vi "ziSaveSettings.vi"(3 "Error In":errorcluster, 4 "Path (\"\")":string, 5 "file path (dialog if empty)":path, 6 "Handle In":T1 {"Handle" format="0x%08x"; "Conn" format="0x%08x"}) -> (0 "Error Out":errorcluster, 1 "Saved Array":string[][](array[string]), 2 "Handle Out":T1 {"Handle" format="0x%08x"; "Conn" format="0x%08x"})   [LabVIEW 2009, in "Zurich Instruments LabOne.lvlib"]
uses:
  <instrlib>/Zurich Instruments LabOne/Zurich Instruments LabOne.lvlib
  <instrlib>/Zurich Instruments LabOne/Public/ziTypeHandle.ctl
  <vilib>/regexp/Match Regular Expression.xnode
  <vilib>/Utility/file.llb/Write To Spreadsheet File (string).vi
panel:
  out "node_paths":string[](array[string])
  out "node_values":string[](array[string])
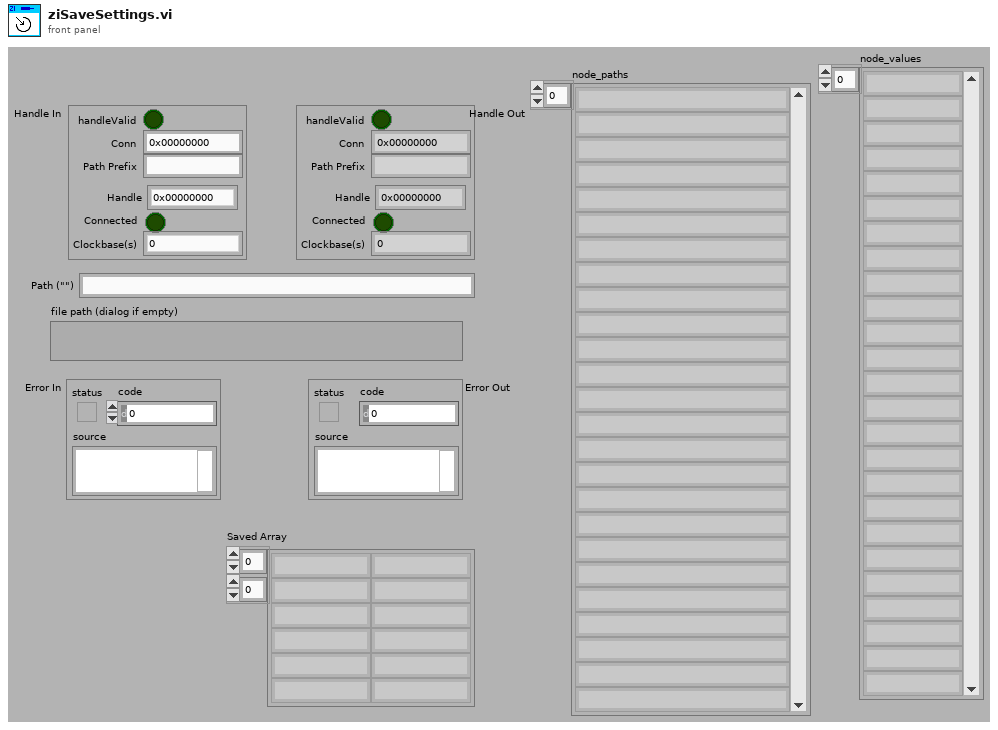
[diagram p1: front panel]
types:
  T1 = typedef "Zurich Instruments LabOne.lvlib/ziTypeHandle.ctl" = cluster{"handleValid":bool, "Conn":u64, "Path Prefix":string, "Handle":u64, "Connected":bool, "Clockbase(s)":dbl}
  T2 = cluster{"Recursive":bool, "Absolut":bool, "Leafs Only":bool, "Settings Only":bool}
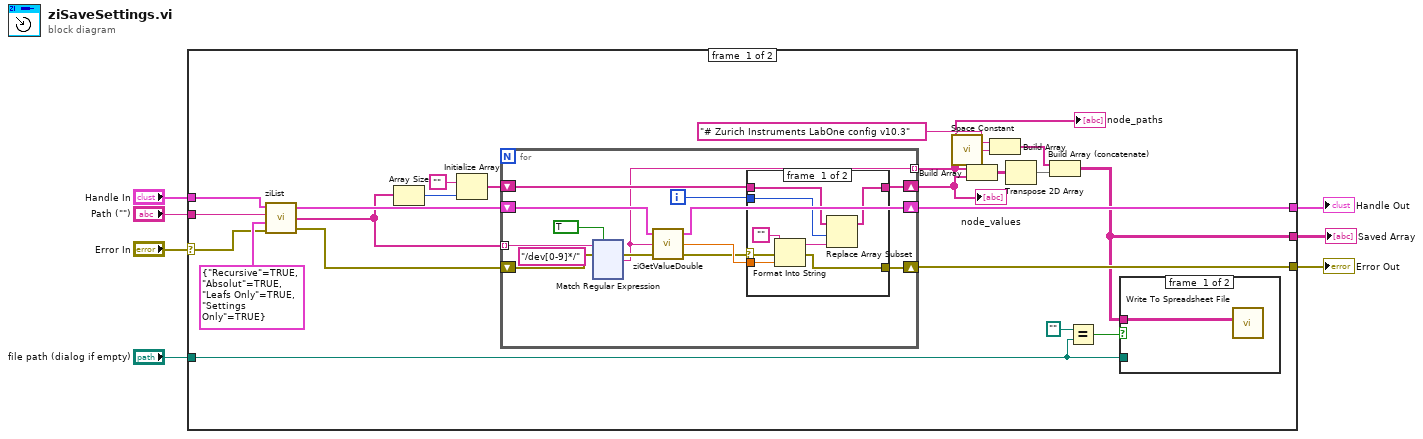
[diagram p0: block diagram]
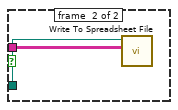
[diagram p2: hidden frame]
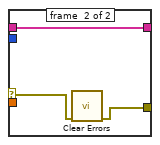
[diagram p3: hidden frame]
diagram:
  n1 = case shown="No Error" "Error In" {
    selector: "Error In" -> [w8 w165]
    tunnel: [w28 w166] -> w7
    tunnel: [w27 w165] -> w6
    tunnel: "file path (dialog if empty)" -> [w11 _]
    tunnel: "Handle In" -> [w25 w166]
    tunnel: "Path (\"\")" -> [w24 _]
    tunnel: [w15 _] -> w2
    frame #0 {
      n2 = call <instrlib>:"ziList.vi"("Error In"=w8, "Flags (None)"=T2 {"Recursive"=TRUE, "Absolut"=TRUE, "Leafs Only"=TRUE, "Settings Only"=TRUE}, "Path (\"\")"=w24, "Handle In"=w25) -> ("Error Out"=w29:errorcluster, "Nodes"=w13:string[], "Handle Out"=w30:T1)
      n3 = Array Size(array=w13) -> (size(s)=w20:i32)
      n4 = Initialize Array("", w20) -> (w19:string[])
      n5 = for {
        shift-right: [w42] -> w27
        shift-left: w29 -> [w45]
        shift-right: [w44] -> w28
        shift-left: w30 -> [w46]
        tunnel: w13 -> [w38] mode=indexing
        shift-right: [w40] -> w26
        shift-left: w19 -> [w41]
        tunnel: [w36] -> w12 mode=indexing
        i -> [w39]
        n6 = xnode "Match Regular Expression"("input string"=w38, "regular expression"="/dev[0-9]*/", "ignore case? (F)"=TRUE) -> ("after match"=w36:string)  [unwired: 3 in, 4 out]
        n7 = call <instrlib>:"ziGetValueDouble.vi"("error in"=w45, "Path"=w36, "Handle in"=w46) -> ("error out"=w35:errorcluster, "Value"=w43:dbl, "Handle out"=w44:T1)
        n8 = case shown="No Error" w35 {
          selector: w35 -> [w47 w55]
          tunnel: w43 -> [w54 _]
          tunnel: [w53 w56] -> w42
          tunnel: w41 -> [w51 w57]
          tunnel: [w50 w57] -> w40
          tunnel: w39 -> [w48 _]
          frame #0 {
            n9 = Format Into String(initial string="", error in=w47, w54) -> (resulting string=w52:string, error out=w53:errorcluster)  [unwired: 1 in]
            n10 = Replace Array Subset(array=w51, new element=w52, index=w48) -> (w50:string[])
          }
          frame #1 {
            n11 = call <vilib>:"Clear Errors.vi"("error in (no error)"=w55) -> ("error out"=w56:errorcluster)  [unwired: 6 in]
          }
        }
      }
      "node_values" <- w26
      "node_paths" <- w12
      n12 = call <vilib>:"Space Constant.vi"() -> ("String"=w21:string)
      n13 = Build Array(w12, w26) -> (w18:string[][])
      n14 = Build Array("# Zurich Instruments LabOne config v10.3" ("new element/subarray"), w21) -> (w17:string[])
      n15 = Transpose 2D Array(2D array=w18) -> (transposed array=w16:string[][])
      n16 = Build Array (concatenate)(w17, w16) -> (w15:string[][])
      n17 = Equal?(x=path "", y=w11) -> (x = y?=w10:bool)
      n18 = case shown="True" w10 {
        tunnel: w15 -> [w31 w33]
        tunnel: w11 -> [_ w32]
        frame #0 {
          n19 = call-poly <vilib>:"Write To Spreadsheet File.vi"("2D data"=w31) -> ()  [unwired: 7 in, 1 out]
        }
        frame #1 {
          n20 = call-poly <vilib>:"Write To Spreadsheet File.vi"("2D data"=w33, "file path (dialog if empty)"=w32) -> ()  [unwired: 6 in, 1 out]
        }
      }
    }
    frame #1 {
    }
  }
  "Handle Out" <- w7
  "Error Out" <- w6
  "Saved Array" <- w2
